vi "Finish.vi"   [LabVIEW 2020]
doc: "This VIcloses device references, sends final commands to the network tables and the joysticks, and terminates all command and control loops."
uses:
  refnums.vi
  <vilib>/Rock Robotics/WPI/Utilities/WPI_GetSetVariantRefNum.vi
types:
  T1 = typedef "WPI_MotorControlDeviceRef.ctl" = cluster{"DeviceStatus":errorcluster, "Type":T2, "PWM":cluster{"PWM Channel":T3, "DeadBand":T4}, "CAN":cluster{"Device Number":u8, "SetOutput VI Ref":variant, "GetOutput VI Ref":variant, "Enable VI Ref":variant, "Disable VI Ref":variant, "Data":variant}, "Invert":bool, "DIO PWM":cluster{"PWM \"Enable\" Channel":T3, "DIOChannel":T5, "PWM Rate":dbl}}
  T2 = typedef "WPI_MotorControlType.ctl" = enum16{"PWM", "CAN", "DIO PWM"}
  T3 = typedef "FPGA_DIOPWMChannel.ctl" = enum8{"PWM 0", "PWM 1", "PWM 2", "PWM 3", "PWM 4", "PWM 5", "PWM 6", "PWM 7", "PWM 8", "PWM 9", "PWM MXP 0", "PWM MXP 1", "PWM MXP 2", "PWM MXP 3", "PWM MXP 4", "PWM MXP 5", "PWM MXP 6", "PWM MXP 7", "PWM MXP 8", "PWM MXP 9", "Invalid"}
  T4 = typedef "WPI_PWMDeadband.ctl" = cluster{"Name":string, "maxPositivePwm":i32, "minPositivePwm":i32, "centerPwm":i32, "maxNegativePwm":i32, "minNegativePwm":i32, "angularRange":u16}
  T5 = typedef "FPGA_DIOChannel.ctl" = enum8{"DIO 0", "DIO 1", "DIO 2", "DIO 3", "DIO 4", "DIO 5", "DIO 6", "DIO 7", "DIO 8", "DIO 9", "DIO MXP 0", "DIO MXP 1", "DIO MXP 2", "DIO MXP 3", "DIO MXP 4", "DIO MXP 5", "DIO MXP 6", "DIO MXP 7", "DIO MXP 8", "DIO MXP 9", "DIO MXP 10", "DIO MXP 11", "DIO MXP 12", "DIO MXP 13", "DIO MXP 14", "DIO MXP 15", "SPI Port CS1", "SPI Port CS2", "SPI Port CS3", "SPI Port MISO", "SPI Port MOSI", "Invalid"}
  T6 = typedef "WPI_SolenoidDevRef.ctl" = cluster{"DevStatus":errorcluster, "Pneumatics Control Module":u8, "Forward Solenoid Channel":T7, "Reverse Solenoid Channel":T7}
  T7 = typedef "WPI_SolenoidChannel.ctl" = enum8{"Solenoid 0", "Solenoid 1", "Solenoid 2", "Solenoid 3", "Solenoid 4", "Solenoid 5", "Solenoid 6", "Solenoid 7", "Solenoid 8", "Solenoid 9", "Solenoid 10", "Solenoid 11", "Solenoid 12", "Solenoid 13", "Solenoid 14", "Solenoid 15", "Invalid"}
  T8 = typedef "WPI_JoystickDevRef.ctl" = cluster{"Device":T9}
  T9 = typedef "WPI_JoystickDeviceEnum.ctl" = enum16{"USB 0", "USB 1", "USB 2", "USB 3", "USB 4", "USB 5"}
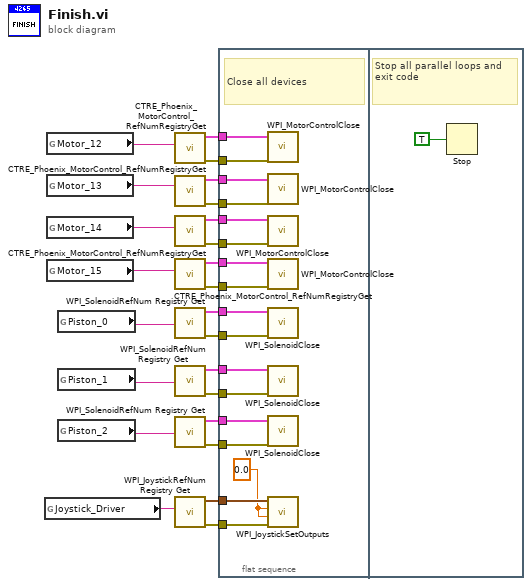
[diagram p0: block diagram]
diagram:
  n1 = global read "refnums.vi" "Joystick_Driver"() -> (w22:string)
  n2 = global read "refnums.vi" "Motor_12"() -> (w21:string)
  n3 = global read "refnums.vi" "Motor_13"() -> (w20:string)
  n4 = global read "refnums.vi" "Motor_14"() -> (w19:string)
  n5 = global read "refnums.vi" "Motor_15"() -> (w18:string)
  n6 = global read "refnums.vi" "Piston_0"() -> (w7:string)
  n7 = global read "refnums.vi" "Piston_1"() -> (w8:string)
  n8 = global read "refnums.vi" "Piston_2"() -> (w9:string)
  n9 = call <vilib>:"CTRE_Phoenix_MotorControl_RefNumRegistryGet.vi"("refnum name"=w21) -> ("error out"=w13:errorcluster, "PhoenixMotorControlDevRef"=w17:T1)  [unwired: 9 in]
  n10 = call <vilib>:"CTRE_Phoenix_MotorControl_RefNumRegistryGet.vi"("refnum name"=w20) -> ("error out"=w12:errorcluster, "PhoenixMotorControlDevRef"=w16:T1)  [unwired: 9 in]
  n11 = call <vilib>:"CTRE_Phoenix_MotorControl_RefNumRegistryGet.vi"("refnum name"=w19) -> ("error out"=w11:errorcluster, "PhoenixMotorControlDevRef"=w15:T1)  [unwired: 9 in]
  n12 = call <vilib>:"CTRE_Phoenix_MotorControl_RefNumRegistryGet.vi"("refnum name"=w18) -> ("error out"=w10:errorcluster, "PhoenixMotorControlDevRef"=w14:T1)  [unwired: 9 in]
  n13 = call <vilib>:"WPI_SolenoidRefNum Registry Get.vi"("refnum name"=w7) -> ("error out"=w5:errorcluster, "SolenoidDevRef"=w6:T6)  [unwired: 9 in]
  n14 = call <vilib>:"WPI_SolenoidRefNum Registry Get.vi"("refnum name"=w8) -> ("error out"=w3:errorcluster, "SolenoidDevRef"=w4:T6)  [unwired: 9 in]
  n15 = call <vilib>:"WPI_SolenoidRefNum Registry Get.vi"("refnum name"=w9) -> ("error out"=w1:errorcluster, "SolenoidDevRef"=w2:T6)  [unwired: 9 in]
  n16 = call <vilib>:"WPI_JoystickRefNum Registry Get.vi"("refnum name"=w22) -> ("error out"=w23:errorcluster, "JoystickDevRef"=w24:T8)  [unwired: 9 in]
  n17 = flat-sequence {
    tunnel: w24 -> [w41]
    tunnel: w23 -> [w40]
    tunnel: w17 -> [w39]
    tunnel: w16 -> [w38]
    tunnel: w15 -> [w37]
    tunnel: w14 -> [w36]
    tunnel: w13 -> [w35]
    tunnel: w12 -> [w34]
    tunnel: w11 -> [w33]
    tunnel: w10 -> [w32]
    tunnel: w6 -> [w31]
    tunnel: w5 -> [w30]
    tunnel: w4 -> [w29]
    tunnel: w3 -> [w28]
    tunnel: w2 -> [w27]
    tunnel: w1 -> [w26]
    frame #0 {
      w25 = sgl 0.0 ("Left Rumble")
      # "Close all devices"
      n18 = call <vilib>:"WPI_MotorControlClose.vi"("error in"=w35, "MotorControlDevRef"=w39) -> ()  [unwired: 9 in, 1 out]
      n19 = call <vilib>:"WPI_MotorControlClose.vi"("error in"=w34, "MotorControlDevRef"=w38) -> ()  [unwired: 9 in, 1 out]
      n20 = call <vilib>:"WPI_MotorControlClose.vi"("error in"=w33, "MotorControlDevRef"=w37) -> ()  [unwired: 9 in, 1 out]
      n21 = call <vilib>:"WPI_MotorControlClose.vi"("error in"=w32, "MotorControlDevRef"=w36) -> ()  [unwired: 9 in, 1 out]
      n22 = call <vilib>:"WPI_SolenoidClose.vi"("error in (no error)"=w30, "SolenoidDevRef"=w31) -> ()  [unwired: 9 in, 1 out]
      n23 = call <vilib>:"WPI_SolenoidClose.vi"("error in (no error)"=w28, "SolenoidDevRef"=w29) -> ()  [unwired: 9 in, 1 out]
      n24 = call <vilib>:"WPI_SolenoidClose.vi"("error in (no error)"=w26, "SolenoidDevRef"=w27) -> ()  [unwired: 9 in, 1 out]
      n25 = call <vilib>:"WPI_JoystickSetOutputs.vi"("error in (no error)"=w40, "Right Rumble"=w25, "Left Rumble"=w25, "JoystickDevRef"=w41) -> ()  [unwired: 6 in, 2 out]
    }
    frame #1 {
      # "Stop all parallel loops and exit code"
      n26 = Stop(stop? (T)=TRUE ("Quit")) -> ()
    }
  }
